vi "close.vi"(8 "error in":errorcluster, 11 "TDMS datalogger runtime in":refnum<class "TDMS datalogger runtime.lvclass">) -> (0 "error out":errorcluster)   [LabVIEW 2013, in "TDMS datalogger runtime.lvclass"]
doc: "Provides an interface for terminating a module instance. While this interface performs no operations, a child should close and deallocate any open references or memory."
uses:
  TDMS datalogger runtime.lvclass
  control enum.ctl
  TDMS datalogger runtime.lvclass/TDMS datalogger runtime.ctl
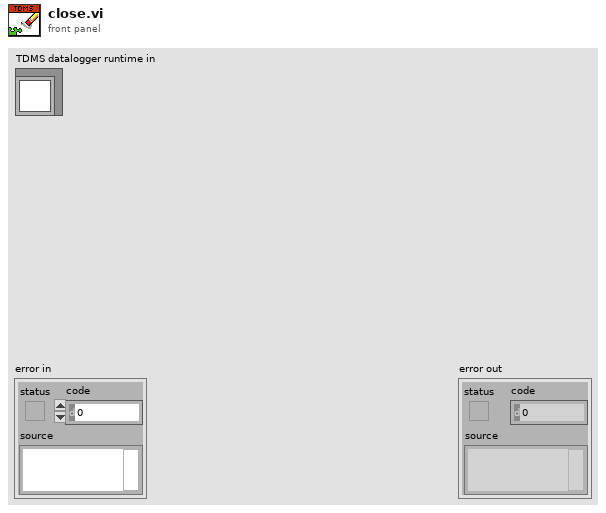
[diagram p1: front panel]
types:
  T1 = typedef "TDMS datalogger runtime.lvclass/control enum.ctl" = enum16{"exit"}
  T2 = typedef "TDMS datalogger runtime.lvclass/sample queue.ctl" = cluster{"data to processor":refnum<queue>, "time to processor":refnum<queue>}
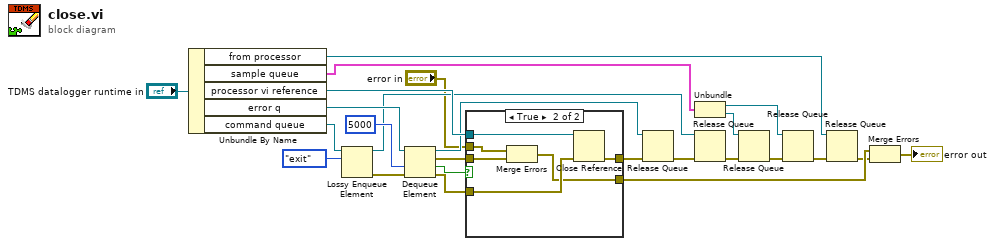
[diagram p0: block diagram]
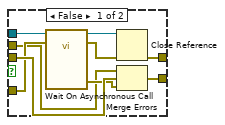
[diagram p2: hidden frame]
diagram:
  n1 = Unbundle By Name("TDMS datalogger runtime in") -> ("from processor"=w15:refnum<queue>, "sample queue"=w19:T2, "processor vi reference"=w21:refnum<vi>, "error q"=w25:refnum<queue>, "command queue"=w9:refnum<queue>)
  n2 = Lossy Enqueue Element(queue=w9, element=control_enum."exit") -> (queue out=w7:refnum<queue>, error out=w2:errorcluster)  [unwired: 1 in, 2 out]
  n3 = Dequeue Element(queue=w25, timeout in ms (-1)=5000, error in (no error)=w2) -> (queue out=w17:refnum<queue>, element=w20:errorcluster, timed out?=w23:bool, error out=w22:errorcluster)
  n4 = case shown="True" w23 {
    tunnel: w22 -> [w28 w38]
    tunnel: w21 -> [w29 w39]
    tunnel: w20 -> [w34 w40]
    tunnel: [w33 w36] -> w14
    tunnel: [w32 w37] -> w18
    tunnel: "error in" -> [w26 w35]
    frame False {
      n5 = call-by-ref "Wait On Asynchronous Call"(reference=w29, error in=w28) -> (reference out=w31:refnum<vi>, error out=w30:errorcluster, 19:"error out"=w27:errorcluster)  [unwired: 19 in]
      n6 = Close Reference(reference=w31, error in (no error)=w30) -> (error out=w32:errorcluster)
      n7 = Merge Errors(w26, w34, w27) -> (w33:errorcluster)
    }
    frame True {
      n8 = Merge Errors(w35, w40) -> (w36:errorcluster)
      n9 = Close Reference(reference=w39, error in (no error)=w38) -> (error out=w37:errorcluster)
    }
  }
  n10 = Release Queue(queue=w17, error in (no error)=w18) -> (error out=w10:errorcluster)  [unwired: 1 in, 2 out]
  n11 = Unbundle(w19) -> ("data to processor"=w4:refnum<queue>, "time to processor"=w3:refnum<queue>)
  n12 = Release Queue(queue=w7, error in (no error)=w10) -> (error out=w6:errorcluster)  [unwired: 1 in, 2 out]
  n13 = Release Queue(queue=w3, error in (no error)=w6) -> (error out=w5:errorcluster)  [unwired: 1 in, 2 out]
  n14 = Release Queue(queue=w4, error in (no error)=w5) -> (error out=w16:errorcluster)  [unwired: 1 in, 2 out]
  n15 = Release Queue(queue=w15, error in (no error)=w16) -> (error out=w13:errorcluster)  [unwired: 1 in, 2 out]
  n16 = Merge Errors(w14, w13) -> (→"error out":errorcluster)
